vi "Leer ultimo valor TDMS.vi"(9 "canal":string, 10 "grupo":string, 11 "file path":path) -> (3 "Value":dbl format="%#_2g")   [LabVIEW 2015]
panel:
  in  "error in":errorcluster
  out "error out":errorcluster
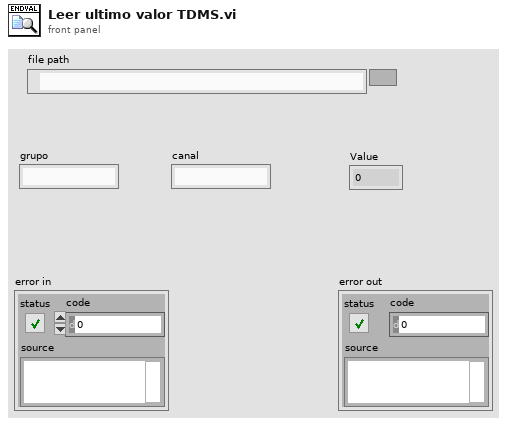
[diagram p1: front panel]
types:
  T1 = enum16{"open", "open or create", "create or replace", "create", "open (read-only)"}
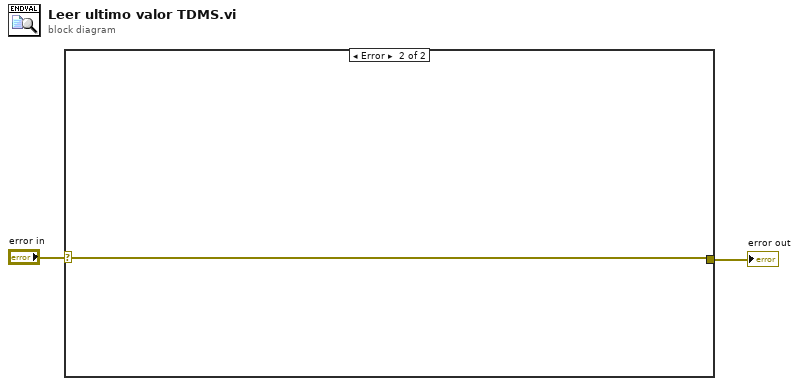
[diagram p0: block diagram]
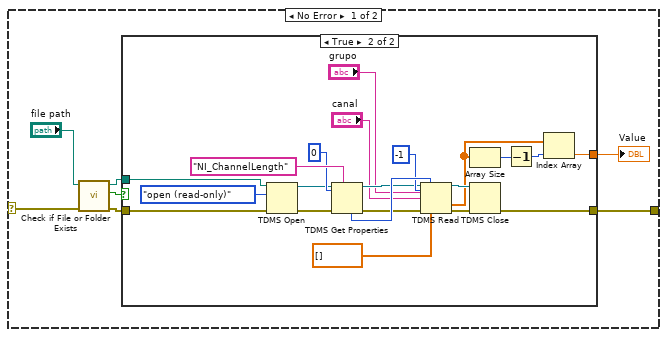
[diagram p2: hidden frame]
diagram:
  n1 = case shown="Error" "error in" {
    selector: "error in" -> [w3 w32]
    tunnel: [w9 w32] -> w2
    frame No Error {
      n2 = call <vilib>:"Check if File or Folder Exists.vi"("error in (no error)"=w3, "path"="file path") -> ("error out"=w8:errorcluster, "file or folder exists?"=w6:bool, "dup path"=w5:path)  [unwired: 7 in]
      n3 = case shown="True" w6 {
        tunnel: [w10 w22] -> w9
        tunnel: w8 -> [w10 w18]
        tunnel: w5 -> [_ w17]
        tunnel: [_ w14] -> w4
        frame False {
        }
        frame True {
          n4 = TDMS Open(8:w18, 10:T1."open (read-only)" ("operation (0:open)"), 11:w17) -> (0:w20:errorcluster, 3:w19:refnum<k34>)  [unwired: 4 in]
          n5 = TDMS Get Properties(5:0, 7:"NI_ChannelLength" ("property name"), 8:w20, 11:w19) -> (0:w27:errorcluster, 3:w26:refnum<k34>, 4:w29:i32)  [unwired: 2 in, 3 out]
          n6 = TDMS Read(0:w26, 1:w29, 2:i64 -1 ("count (-1: all)"), 5:"grupo", 7:"canal", 11:w27, 12:dbl[] []) -> (4:w24:refnum<k34>, 10:w15:dbl[], 15:w23:errorcluster)  [unwired: 1 in, 3 out]
          n7 = Array Size(array=w15) -> (size(s)=w12:i32)
          n8 = TDMS Close(8:w23, 11:w24) -> (0:w22:errorcluster)  [unwired: 1 out]
          n9 = Decrement(x=w12) -> (x-1=w11:i32)
          n10 = Index Array(array=w15, index=w11) -> (element=w14:dbl)
        }
      }
      "Value" <- w4
    }
    frame Error {
    }
  }
  "error out" <- w2
